vi "Quizz10.vi"() -> ()   [LabVIEW 2017]
panel:
  out "result":i8
  out "Boolean":bool
  out "Round LED Blink":i32
  out "AVG":i8
  out "Array":dbl[](array[numeric])
  # "ทศนิยมปัดขึ้น"
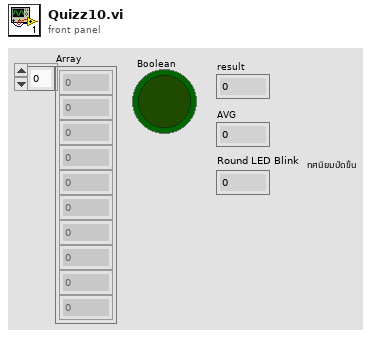
[diagram p1: front panel]
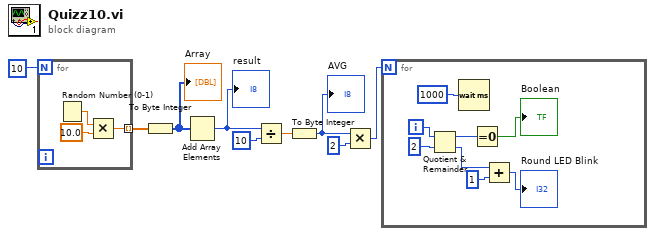
[diagram p0: block diagram]
diagram:
  n1 = for {
    N: 10 -> [_]
    tunnel: [w10] -> w8 mode=indexing
    n2 = Random Number (0-1)() -> (number: 0 to 1=w12:dbl)
    n3 = Multiply(x=w12, y=10.0) -> (x*y=w10:dbl)
  }
  n4 = To Byte Integer(number=w8) -> (8bit integer=w5:i8[])
  "Array" <- w5
  n5 = Add Array Elements(numeric array=w5) -> (sum=w4:i8)
  "result" <- w4
  n6 = Divide(x=w4, y=i8 10) -> (x/y=w6:dbl)
  n7 = To Byte Integer(number=w6) -> (8bit integer=w2:i8)
  "AVG" <- w2
  n8 = Multiply(x=w2, y=i8 2) -> (x*y=w3:i8)
  n9 = for {
    N: w3 -> [_]
    i -> [w19]
    n10 = Quotient & Remainder(x=w19, y=2) -> (x-y*floor(x/y)=w14:i32, floor(x/y)=w17:i32)
    n11 = Wait (ms)(milliseconds to wait=u32 1000) -> ()  [unwired: 1 out]
    n12 = Equal To 0?(x=w14) -> (x = 0?=→"Boolean":bool)
    n13 = Add(x=w17, y=1) -> (x+y=→"Round LED Blink":i32)
  }
